vi "Post_Process_Raw_data.vi"(0 "Select Plug Ins":bool, 2 "Post processed Results folder":path, 3 "No dialogs":bool, 5 "Save results to":T1(ring)=enum."Original Results Filenames with _PP", 11 "Selected files":path[](array[path]), 12 "Current Results filenames":path[](array[path]), 13 "Results Plotter Rows":string[][](array[string])) -> (15 "Post processed Results folder Out":path)   [LabVIEW 2013]
uses:
  Anemometry Sub Vis/Controls/File_Selector_Type.ctl
  Anemometry Sub Vis/Controls/Setup.ctl
  Anemometry Sub Vis/Controls/Post_Process.ctl
  Anemometry Sub Vis/Controls/Save_Data.ctl
  Anemometry Sub Vis/Globals/Meas_global.vi
  Anemometry Sub Vis/Globals/Plug_in_data_global.vi
panel:
  out "Single Filename":string
  out "Files not found":i32
  out "Files not Found":path[](array[path])
  out "Checking":i32
  in  "Previous Choice":path
  in  "Search String":string
  in  "Boolean":bool
  in  "Pause Mode":enum16{"Continuous Running", "After Each File"}(ring)
  in  "At Dialog Prompt Post Process":T2=enum."All files listed in selected file"
  out "Files Processed":i32(slide) scale=0.0..253.0
  in  "stop":bool
  out "Files To Process":path[](array[path])
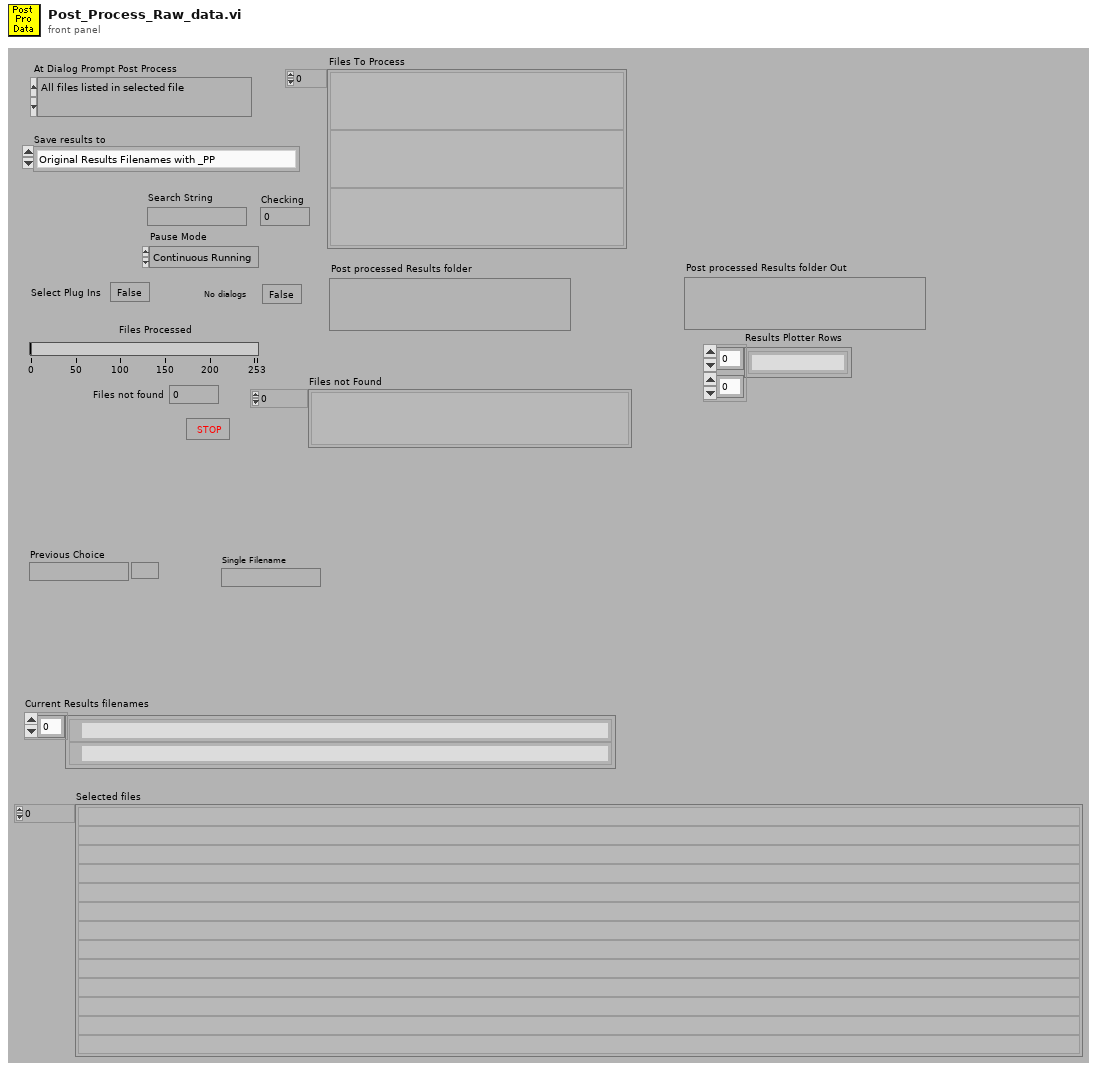
[diagram p1: front panel]
types:
  T1 = enum16{"A single file", "Original Results Filenames with _PP", "Current Results Filenames"}
  T2 = typedef "File_Selector_Type.ctl" = enum16{"The Selected File", "The Selected Folder", "Files containing the search string in the selected folder", "All files listed in selected file"}
  T3 = typedef "Setup.ctl" = enum16{"Run Program", "Show Setup", "Save Current Setup", "Setup Front Panel"}
  T4 = typedef "Save_Data.ctl" = enum16{"Save No Data", "Save Data"}
  T5 = typedef "Post_Process.ctl" = enum16{"Take New Data", "Post Process Raw Data File"}
  T6 = enum16{"Left Button", "Center Button", "Right Button", "Window Close"}
  T7 = typedef "Multi_Run_Status.ctl" = enum16{"Continue", "Jump to Next Point", "Jump to Next Row", "Jump To Fall Back", "Terminate Run"}
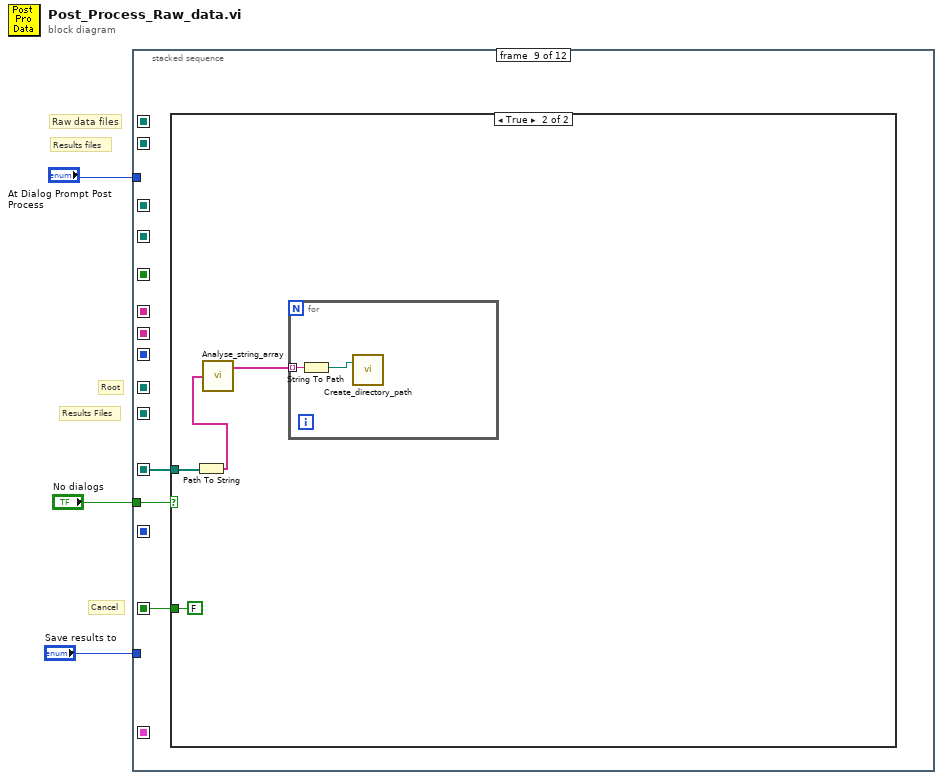
[diagram p0: block diagram]
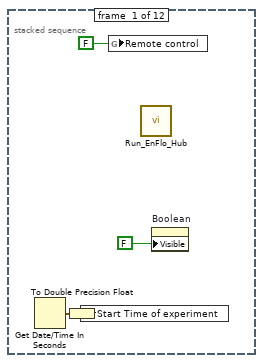
[diagram p2: hidden frame]
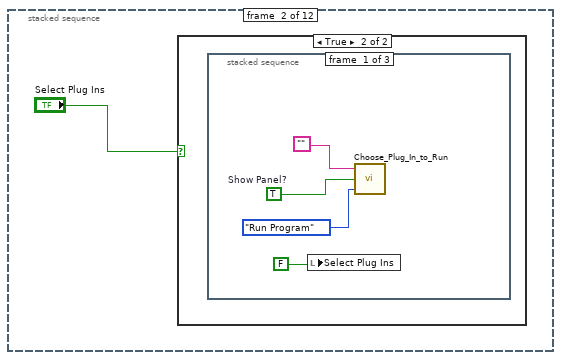
[diagram p3: hidden frame]
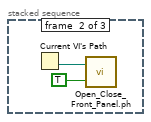
[diagram p5: hidden frame]
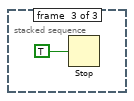
[diagram p6: hidden frame]
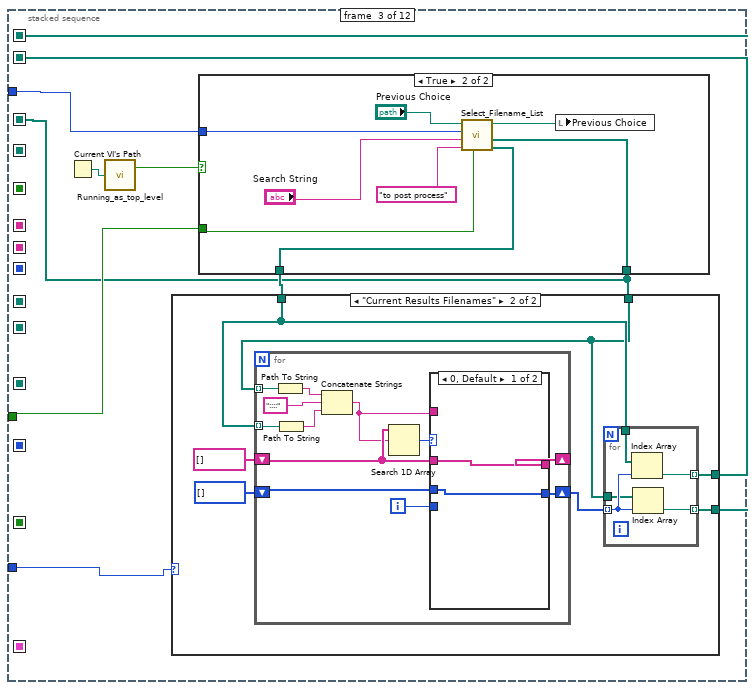
[diagram p7: hidden frame]
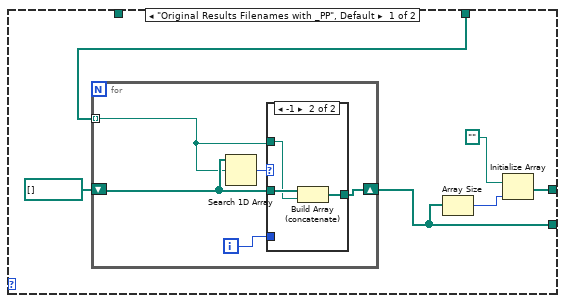
[diagram p8: hidden frame]
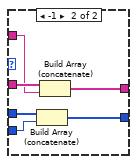
[diagram p10: hidden frame]
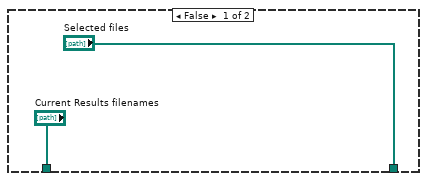
[diagram p11: hidden frame]
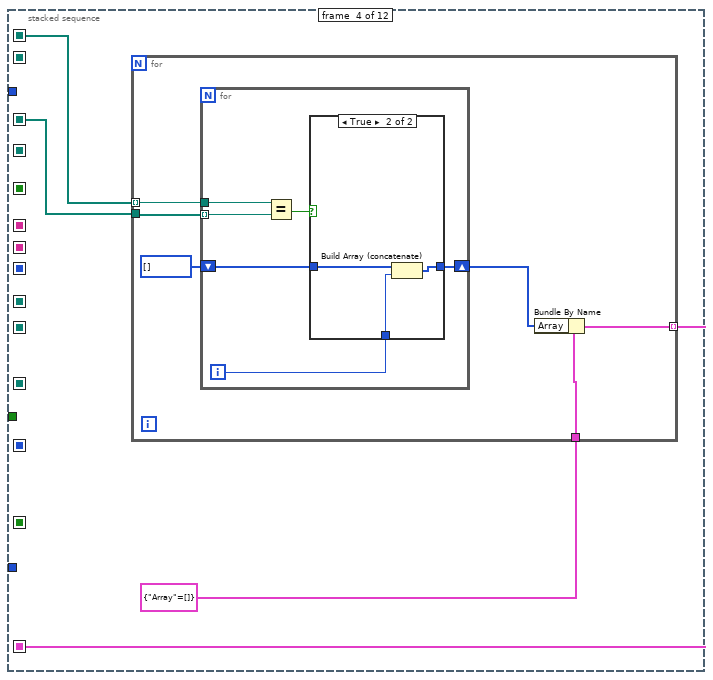
[diagram p12: hidden frame]
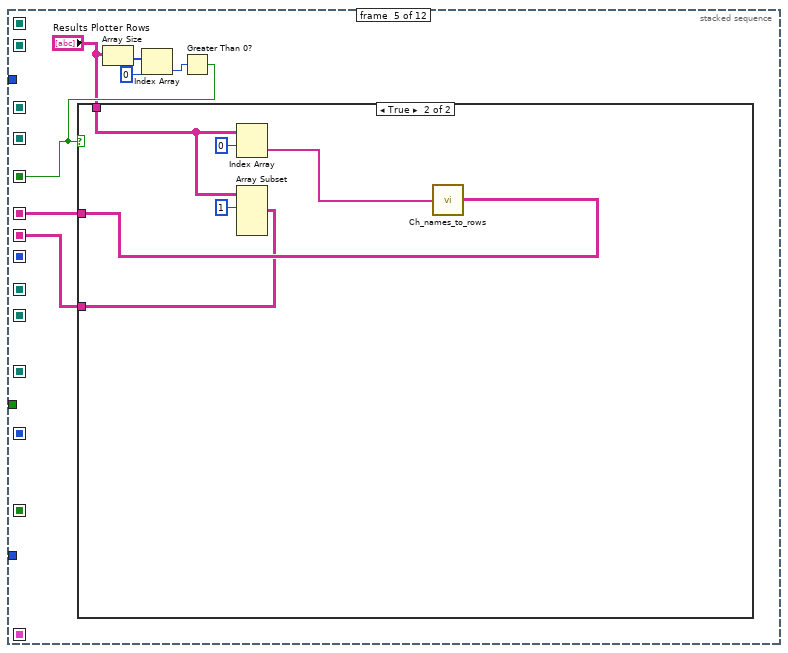
[diagram p14: hidden frame]
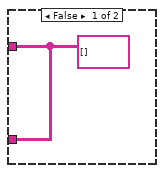
[diagram p15: hidden frame]
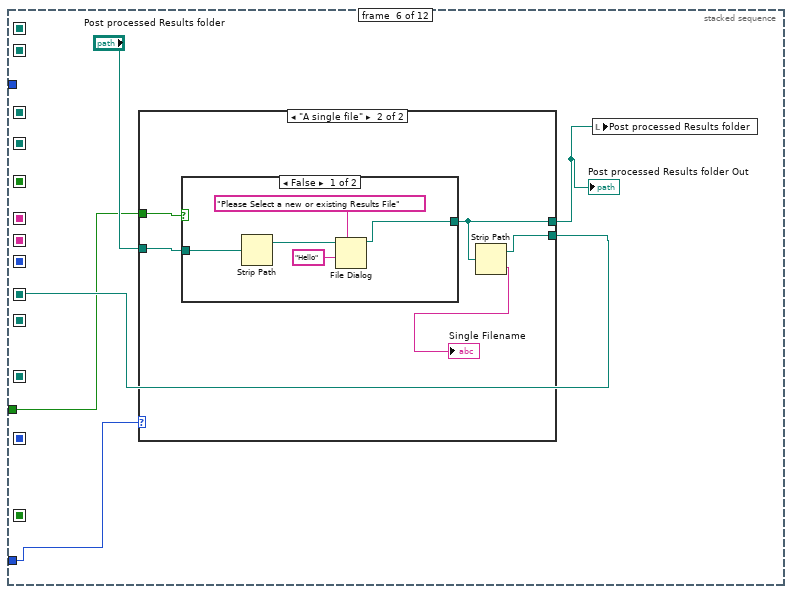
[diagram p16: hidden frame]
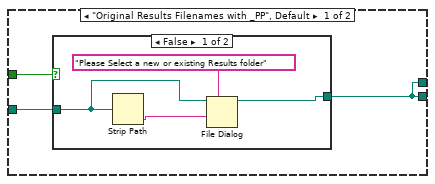
[diagram p17: hidden frame]
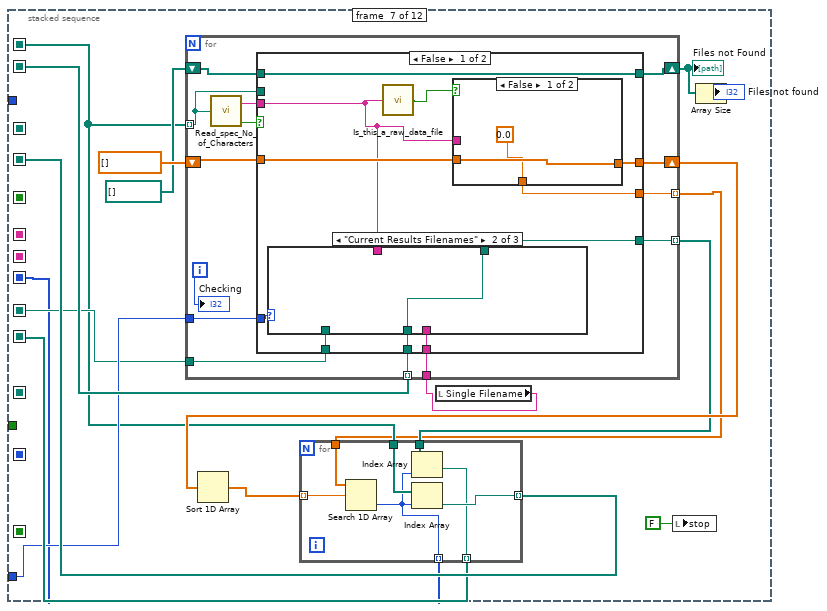
[diagram p20: hidden frame]
diagram:
  # "Cancel"
  # "Results files"
  # "Raw data files"
  # "Root"
  # "Results Files"
  n1 = stacked-sequence {
    seq-local: [_ _ _ _ _ _ w153 _ _ _ _ _] -> [_ _ _ _ _ _ _ _ _ w283 w297 _]
    seq-local: [_ _ _ _ _ _ _ _ _ w288 _ _] -> [_ _ _ _ _ _ _ _ _ _ w296 _]
    seq-local: [_ _ w18 _ _ _ _ _ _ _ _ _] -> [_ _ _ w84 _ _ w142 _ _ _ _ _]
    seq-local: [_ _ _ _ _ w120 _ _ _ _ _ _] -> [_ _ _ _ _ _ w145 w212 _ _ _ _]
    seq-local: [_ _ _ _ _ _ w151 _ _ _ _ _] -> [_ _ _ _ _ _ _ w215 _ _ _ _]
    seq-local: [_ _ _ _ _ _ _ w211 _ _ _ _] -> [_ _ _ _ _ _ _ _ w255 _ w295 w368]
    seq-local: [_ _ w19 _ _ _ _ _ _ _ _ _] -> [_ _ _ _ _ _ w147 _ _ _ _ _]
    seq-local: [_ _ _ _ w108 _ _ _ _ _ _ _] -> [_ _ _ _ _ _ _ _ _ _ w294 _]
    seq-local: [_ _ _ _ w107 _ _ _ _ _ _ _] -> [_ _ _ _ _ _ _ _ _ _ w291 _]
    seq-local: [_ _ _ _ w103 _ _ _ _ _ _ _] -> [_ _ _ _ _ _ _ _ _ _ w293 _]
    seq-local: [_ _ _ _ _ _ w143 _ _ _ _ _] -> [_ _ _ _ _ _ _ _ _ _ w292 _]
    seq-local: [_ _ _ w82 _ _ _ _ _ _ _ _] -> [_ _ _ _ _ _ _ _ _ _ w290 _]
    seq-local: [_ _ w16 _ _ _ _ _ _ _ _ _] -> [_ _ _ w85 _ _ _ _ _ _ _ _]
    seq-local: [_ _ _ _ _ _ _ _ w254 _ _ _] -> [_ _ _ _ _ _ _ _ _ _ w289 _]
    tunnel: "At Dialog Prompt Post Process" -> [_ _ w24 _ _ _ _ _ _ _ _ _]
    tunnel: "No dialogs" -> [_ _ w23 _ _ w118 _ _ w256 _ _ _]
    tunnel: "Save results to" -> [_ _ w17 _ _ w117 w146 w214 _ _ _ _]
    frame #0 {
      n2 = Get Date/Time In Seconds() -> (seconds since 1Jan1904=w4:timestamp)
      n3 = To Double Precision Float(number=w4) -> (double precision float=w5:dbl)
      n4 = global write "Meas_global.vi" "Start Time of experiment"(w5) -> ()
      n5 = global write "Meas_global.vi" "Remote control"(FALSE ("Remote control")) -> ()
      n6 = call "Run_EnFlo_Hub.vi"() -> ()  [unwired: 8 out]
      n7 = property on="Boolean" class="Bool"("Visible"=FALSE ("Write Attribute")) -> ()  [unwired: 2 in, 2 out]
    }
    frame #1 {
      n8 = case shown="True" "Select Plug Ins" {
        frame False {
        }
        frame True {
          n9 = stacked-sequence {
            frame #0 {
              w12 = TRUE  # Show Panel?
              n10 = local write "Select Plug Ins"(FALSE ("Select Local ADAM Channels")) -> ()
              n11 = call "Choose_Plug_In_to_Run.vi"("setup"=Setup."Run Program", "Show Panel?"=w12, "Setup String In"="") -> ()  [unwired: 2 out]
            }
            frame #1 {
              n12 = Current VI's Path() -> (path=w14:path)
              n13 = call "Open_Close_Front_Panel.ph.vi"("Front Panel Window:Open"=TRUE, "VI path"=w14) -> ()  [unwired: 2 out]
            }
            frame #2 {
              n14 = Stop(stop? (T)=TRUE) -> ()
            }
          }
        }
      }
    }
    frame #2 {
      n15 = Current VI's Path() -> (path=w22:path)
      n16 = call "Running_as_top_level.vi"("Vi path name"=w22) -> ("Top Level"=w21:bool)  [unwired: 1 out]
      n17 = case shown="True" w21 {
        tunnel: w24 -> [_ w81]
        tunnel: w23 -> [_ w76]
        tunnel: ["Selected files" w75] -> w16
        tunnel: ["Current Results filenames" w74] -> w20
        frame False {
        }
        frame True {
          n18 = call "Select_Filename_List.vi"("No dialogs"=w76, "File Type"="to post process", "Search String"="Search String", "At Dialog Prompt Post Process"=w81, "Previous Choice"="Previous Choice") -> ("Current Results filenames"=w74:path[], "Selected files"=w75:path[], "Choosen path"=w77:path)  [unwired: 1 out]
          n19 = local write "Previous Choice"(w77) -> ()
        }
      }
      n20 = case shown="\"Current Results Filenames\"" w17 {
        tunnel: w16 -> [w30 w43]
        tunnel: w20 -> [_ w44]
        tunnel: [w26 w42] -> w19
        tunnel: [w28 w41] -> w18
        frame "Original Results Filenames with _PP", Default {
          n21 = for {
            shift-right: [w34] -> w28
            shift-left: path[] [] -> [w35]
            tunnel: w30 -> [w31] mode=indexing
            i -> [w32]
            n22 = Search 1D Array(1D array=w35, element=w31) -> (index of element=w33:i32)  [unwired: 1 out]
            n23 = case shown="-1" w33 {
              tunnel: w35 -> [w36 w39]
              tunnel: [w36 w38] -> w34
              tunnel: w31 -> [_ w37]
              tunnel: w32 -> [_ _]
              frame 0, Default {
              }
              frame -1 {
                n24 = Build Array (concatenate)(w39, w37) -> (w38:path[])
              }
            }
          }
          n25 = Array Size(array=w28) -> (size(s)=w27:i32)
          n26 = Initialize Array(path "", w27) -> (w26:path[])
        }
        frame "Current Results Filenames" {
          n27 = for {
            shift-right: [w62] -> _
            shift-left: string[] [] -> [w63]
            tunnel: w43 -> [w61] mode=indexing
            tunnel: w44 -> [w55] mode=indexing
            shift-right: [w57] -> w40
            shift-left: i32[] [] -> [w56]
            i -> [w58]
            n28 = Path To String(path=w61) -> (string=w60:string)
            n29 = Path To String(path=w55) -> (string=w54:string)
            n30 = Concatenate Strings(w60, "::::" ("string"), w54) -> (w53:string)
            n31 = Search 1D Array(1D array=w63, element=w53) -> (index of element=w52:i32)  [unwired: 1 out]
            n32 = case shown="0, Default" w52 {
              tunnel: w63 -> [w65 w71]
              tunnel: [w65 w70] -> w62
              tunnel: w53 -> [_ w67]
              tunnel: w58 -> [_ w66]
              tunnel: [w64 w69] -> w57
              tunnel: w56 -> [w64 w68]
              frame 0, Default {
              }
              frame -1 {
                n33 = Build Array (concatenate)(w68, w66) -> (w69:i32[])
                n34 = Build Array (concatenate)(w71, w67) -> (w70:string[])
              }
            }
          }
          n35 = for {
            tunnel: w40 -> [w51] mode=indexing
            tunnel: w44 -> [w50]
            tunnel: w43 -> [w49]
            tunnel: [w48] -> w42 mode=indexing
            tunnel: [w47] -> w41 mode=indexing
            n36 = Index Array(array=w50, index=w51) -> (element=w48:path)
            n37 = Index Array(array=w49, index=w51) -> (element=w47:path)
          }
        }
      }
    }
    frame #3 {
      n38 = for {
        tunnel: w85 -> [w90]
        tunnel: w84 -> [w91] mode=indexing
        tunnel: cluster{"Array":i64[]} {"Array"=[]} ("Cluster") -> [w88]
        tunnel: [w86] -> w82 mode=indexing
        n39 = for {
          tunnel: w91 -> [w97]
          tunnel: w90 -> [w96] mode=indexing
          shift-right: [w93] -> w87
          shift-left: i32[] [] -> [w94]
          i -> [w92]
          n40 = Equal?(x=w97, y=w96) -> (x = y?=w95:bool)
          n41 = case shown="True" w95 {
            tunnel: w94 -> [w98 w101]
            tunnel: [w98 w100] -> w93
            tunnel: w92 -> [_ w99]
            frame False {
            }
            frame True {
              n42 = Build Array (concatenate)(w101, w99) -> (w100:i32[])
            }
          }
        }
        n43 = Bundle By Name(cluster=w88, "Array"=w87) -> (w86:cluster{"Array":i64[]})
      }
    }
    frame #4 {
      n44 = Array Size(array="Results Plotter Rows") -> (size(s)=w106:i32[])
      n45 = Index Array(array=w106, index=0) -> (element=w104:i32)
      n46 = Greater Than 0?(x=w104) -> (x > 0?=w103:bool)
      n47 = case shown="True" w103 {
        tunnel: [w109 w115] -> w108
        tunnel: [w109 w110] -> w107
        tunnel: "Results Plotter Rows" -> [_ w113]
        frame False {
          w109 = string[][] [] ("3 Row names")
        }
        frame True {
          n48 = Index Array(array=w113, index (row)=0 ("index")) -> (element=w111:string[])  [unwired: 1 in]
          n49 = Array Subset(array=w113, index (row)=1 ("index")) -> (w110:string[][])  [unwired: 3 in]
          n50 = call "Ch_names_to_rows.vi"("Channel Names"=w111) -> ("3 Row names"=w115:string[][])
        }
      }
    }
    frame #5 {
      n51 = case shown="\"A single file\"" w117 {
        tunnel: [w121 w130] -> w120
        tunnel: "Post processed Results folder" -> [w123 w133]
        tunnel: w118 -> [w122 w132]
        tunnel: [w121 w131] -> w116
        frame "Original Results Filenames with _PP", Default {
          n52 = case shown="False" w122 {
            tunnel: [w127 w128] -> w121
            tunnel: w123 -> [w124 w128]
            frame False {
              n53 = Strip Path(path=w124) -> (name=w125:string)  [unwired: 1 out]
              n54 = File Dialog(7:"Please Select a new or existing Results folder" ("prompt"), 9:w125, 11:w124) -> (3:w127:path)  [unwired: 1 in, 6 out]
            }
            frame True {
            }
          }
        }
        frame "A single file" {
          n55 = case shown="False" w132 {
            tunnel: w133 -> [w137 w139]
            tunnel: [w136 w139] -> w131
            frame False {
              n56 = Strip Path(path=w137) -> (stripped path=w135:path)  [unwired: 1 out]
              n57 = File Dialog(7:"Please Select a new or existing Results File" ("prompt"), 9:"Hello" ("default name"), 11:w135) -> (3:w136:path)  [unwired: 1 in, 6 out]
            }
            frame True {
            }
          }
          n58 = Strip Path(path=w131) -> (stripped path=w130:path, name=→"Single Filename":string)
        }
      }
      "Post processed Results folder Out" <- w116
      n59 = local write "Post processed Results folder"(w116) -> ()
    }
    frame #6 {
      n60 = local read "Single Filename"() -> (w144:string)
      n61 = for {
        tunnel: w142 -> [w172] mode=indexing
        shift-right: [w176] -> w156
        shift-left: dbl[] [] -> [w177]
        shift-right: [w173] -> w149
        shift-left: path[] [] -> [w174]
        tunnel: w147 -> [w169] mode=indexing
        tunnel: w146 -> [w168]
        tunnel: w145 -> [w167]
        tunnel: w144 -> [w166]
        tunnel: [w165] -> w141 mode=indexing
        tunnel: [w164] -> w140 mode=indexing
        i -> [w175]
        n62 = call "Read_spec_No_of_Characters.vi"("Filename"=w172) -> ("character string"=w171:string, "Error?"=w170:bool)
        n63 = case shown="False" w170 {
          tunnel: w177 -> [w188 w210]
          tunnel: [w187 w210] -> w176
          tunnel: w172 -> [_ w208]
          tunnel: w174 -> [w185 w209]
          tunnel: [w185 w207] -> w173
          tunnel: w171 -> [w184 _]
          tunnel: w169 -> [w182 w206]
          tunnel: w168 -> [w183 _]
          tunnel: w167 -> [w181 _]
          tunnel: w166 -> [w180 _]
          tunnel: [w179 w206] -> w165
          tunnel: [w178 0.0 ("Value")] -> w164
          frame False {
            n64 = case shown="\"Current Results Filenames\"" w183 {
              tunnel: [w191 w192 w195] -> w179
              tunnel: w184 -> [_ _ w193]
              tunnel: w182 -> [_ w192 _]
              tunnel: w181 -> [w190 _ _]
              tunnel: w180 -> [w189 _ _]
              frame "A single file" {
                n65 = Build Path(base path=w190, name or relative path=w189) -> (appended path=w191:path)
              }
              frame "Current Results Filenames" {
              }
              frame "Original Results Filenames with _PP" {
                w196 = FALSE  # Show Dialog?
                n66 = call "Get_Characters_from_string.vi"("Show Dialog?"=w196, "Input string"=w193, "Variable name"="Results filename") -> ("Value"=w194:string)  [unwired: 1 out]
                n67 = call "String_to_Pathname.vi"("Input String"=w194) -> ("path"=w195:path)
              }
            }
            n68 = call "Is_this_a_raw_data_file.vi"("character string"=w184) -> ("Raw Dat File?"=w186:bool)  [unwired: 2 out]
            n69 = case shown="False" w186 {
              tunnel: w188 -> [w199 w201]
              tunnel: [w199 w204] -> w187
              tunnel: w184 -> [_ w202]
              tunnel: [0.0 ("Value") w200] -> w178
              frame False {
              }
              frame True {
                n70 = call "Get_value_from_string.vi"("Input string"=w202, "Variable name"="Seconds since 1/1/04") -> ("Value"=w200:dbl)  [unwired: 1 in, 1 out]
                n71 = Build Array (concatenate)(w201, w200) -> (w204:dbl[])
              }
            }
          }
          frame True {
            n72 = Build Array (concatenate)(w209, w208) -> (w207:path[])
          }
        }
        "Checking" <- w175
      }
      "Files not Found" <- w149
      n73 = Sort 1D Array(array=w156) -> (sorted array=w155:dbl[])
      n74 = for {
        tunnel: w140 -> [w163]
        tunnel: w155 -> [w162] mode=indexing
        tunnel: w142 -> [w161]
        tunnel: [w160] -> w153 mode=indexing
        tunnel: w141 -> [w159]
        tunnel: [w158] -> w151 mode=indexing
        tunnel: [w157] -> w143 mode=indexing
        n75 = Search 1D Array(1D array=w163, element=w162) -> (index of element=w157:i32)  [unwired: 1 out]
        n76 = Index Array(array=w159, index=w157) -> (element=w158:path)
        n77 = Index Array(array=w161, index=w157) -> (element=w160:path)
      }
      n78 = local write "stop"(FALSE ("stop")) -> ()
      n79 = Array Size(array=w149) -> (size(s)=→"Files not found":i32)
    }
    frame #7 {
      n80 = case shown="\"Original Results Filenames with _PP\"" w214 {
        tunnel: [FALSE TRUE] -> w213
        tunnel: w214 -> [_ _]
        frame "A single file", Default {
        }
        frame "Original Results Filenames with _PP" {
        }
      }
      n81 = for {
        tunnel: w215 -> [w249] mode=indexing
        tunnel: w213 -> [w221]
        tunnel: w212 -> [w220]
        tunnel: [w218] -> w211 mode=indexing
        w234 = "_" ("Replace with")
        n82 = Strip Path(path=w249) -> (name=w222:string)  [unwired: 1 out]
        n83 = Concatenate Strings("[" ("Substring"), ":", "/", "\\\\", "|", "?", ">", "<", "*", "\"", "]" ("Substring")) -> (w237:string)
        n84 = call <vilib>:"Trim Whitespace.vi"("string"=w222) -> ("trimmed string"=w236:string)  [unwired: 1 in]
        n85 = call "Add_filename_suffix.vi"("Filename"=w236) -> ("Original Suffix"=w226:string, "Base name"=w235:string)  [unwired: 1 in, 2 out]
        n86 = call "Replace_Character.vi"("Replace with"=w234, "Input String"=w235, "Search For"=w237) -> ("Output string"=w230:string)  [unwired: 1 out]
        n87 = call "Replace_Character.vi"("Replace with"="_", "Input String"=w230, "Search For"=" ") -> ("Output string"=w231:string)  [unwired: 1 out]
        n88 = case shown="False" w221 {
          tunnel: [w250 w252] -> w233
          tunnel: w231 -> [w250 w251]
          frame False {
          }
          frame True {
            n89 = Concatenate Strings(w251, "_pp" ("Substring")) -> (w252:string)
          }
        }
        n90 = Empty String/Path?(string/path=w226) -> (empty?=w227:bool)
        n91 = Select(t=".xls", s=w227, f=w226) -> (s? t:f=w225:string)
        n92 = call "Replace_Character.vi"("Replace with"=w234, "Input String"=w233, "Search For"="__") -> ("Output string"=w224:string)  [unwired: 1 out]
        n93 = Concatenate Strings(w224, w225) -> (w219:string)
        n94 = Build Path(base path=w220, name or relative path=w219) -> (appended path=w218:path)
      }
    }
    frame #8 {
      n95 = case shown="True" w256 {
        tunnel: w255 -> [w260 w278]
        tunnel: [w257 FALSE ("stop? (T)")] -> w254
        frame False {
          n96 = Path To String(path=w260) -> (string=w259:string[])
          n97 = call "Analyse_string_array.vi"("String array"=w259) -> ("Unique strings"=w258:string[])  [unwired: 2 out]
          n98 = for {
            tunnel: w258 -> [w263] mode=indexing
            tunnel: [w262] -> w257
            stop <- w262 stop-if-true
            n99 = String To Path(string=w263) -> (path=w261:path)
            n100 = call "Does_file_exist_(simple).vi"("Pathname"=w261) -> ("exists?"=w264:bool)
            n101 = call "Create_directory_path.vi"("Path name"=w261) -> ()  [unwired: 1 in, 2 out]
            n102 = case shown="True" w264 {
              tunnel: w261 -> [_ w267]
              tunnel: [FALSE ("stop? (T)") w266] -> w262
              frame False {
              }
              frame True {
                n103 = Format Into String(format string="%s\nAlready exists. Do you want to overwrite?", w267) -> (resulting string=w270:string)  [unwired: 2 in, 1 out]
                n104 = call <vilib>:"Three Button Dialog.vi"("Allow user to close window? (TRUE)"=FALSE, "message"=w270) -> ("Which Button?"=w268:T6)  [unwired: 9 in]
                n105 = case shown="\"Center Button\"" w268 {
                  tunnel: w267 -> [w273 _ _ _]
                  tunnel: [FALSE ("stop? (T)") FALSE ("stop? (T)") TRUE ("stop? (T)") FALSE ("stop? (T)")] -> w266
                  frame "Left Button" {
                    n106 = Delete(path (use dialog)=w273) -> ()  [unwired: 4 in, 3 out]
                  }
                  frame "Center Button" {
                  }
                  frame "Right Button" {
                  }
                  frame "Window Close" {
                  }
                }
              }
            }
          }
        }
        frame True {
          n107 = Path To String(path=w278) -> (string=w279:string[])
          n108 = call "Analyse_string_array.vi"("String array"=w279) -> ("Unique strings"=w277:string[])  [unwired: 2 out]
          n109 = for {
            tunnel: w277 -> [w282] mode=indexing
            n110 = String To Path(string=w282) -> (path=w281:path)
            n111 = call "Create_directory_path.vi"("Path name"=w281) -> ()  [unwired: 1 in, 2 out]
          }
        }
      }
    }
    frame #9 {
      w284 = 0 ("Files Processed")
      n112 = Array Size(array=w283) -> (size(s)=w288:i32)
      n113 = Array Size(array=w283) -> (size(s)=w286:i32)
      n114 = property on="Files Processed" class="Slide (strict)"("Scale.Range:Minimum"=0.0 ("Write Attribute"), "Scale.Range:Maximum"=w286) -> ()  [unwired: 2 in, 2 out]
      n115 = local write "Files Processed"(w284) -> ()
      n116 = Build Array(w284) -> (w285:i32[])
      n117 = property on="Attribute Node" class="Arr (strict)"("Index Values"=w285) -> ()  [unwired: 2 in, 2 out]
      "Files To Process" <- w283
    }
    frame #10 {
      n118 = case shown="False" w289 {
        tunnel: w297 -> [w305 _]
        tunnel: w296 -> [w304 _]
        tunnel: w295 -> [w303 _]
        tunnel: w294 -> [w302 _]
        tunnel: w293 -> [w301 _]
        tunnel: w292 -> [w300 _]
        tunnel: w291 -> [w299 _]
        tunnel: w290 -> [w298 _]
        frame False {
          n119 = while {
            tunnel: w303 -> [w311] mode=indexing
            tunnel: w304 -> [w314]
            tunnel: w305 -> [w315] mode=indexing
            tunnel: w302 -> [w310]
            tunnel: w300 -> [w307] mode=indexing
            tunnel: w301 -> [w309]
            tunnel: w299 -> [w308]
            tunnel: w298 -> [w306]
            i -> [w313]
            stop <- w312 continue-if-true
            n120 = stacked-sequence {
              seq-local: [_ w337 _ _] -> [_ _ w341 _]
              tunnel: w311 -> [_ w339 _ _]
              tunnel: w315 -> [_ w338 _ _]
              tunnel: w314 -> [_ _ w343 _]
              tunnel: w313 -> [_ _ w342 w365]
              tunnel: [_ _ w340 _] -> w312
              tunnel: w310 -> [w324 _ _ _]
              tunnel: w309 -> [w323 _ _ _]
              tunnel: w308 -> [w319 _ _ _]
              tunnel: w307 -> [w320 _ _ _]
              tunnel: w306 -> [w321 _ _ _]
              frame #0 {
                n121 = Index Array(array=w321, index=w320) -> (element=w318:cluster{"Array":i64[]})
                n122 = Unbundle By Name(w318) -> ("Array"=w317:i64[])
                n123 = for {
                  tunnel: w319 -> [w327]
                  tunnel: w317 -> [w326] mode=indexing
                  tunnel: [w325] -> w316 mode=indexing
                  n124 = Index Array(array=w327, index (row)=w326) -> (element=w325:string[])  [unwired: 1 in]
                }
                n125 = case shown="True" w323 {
                  tunnel: w324 -> [_ w331]
                  tunnel: w316 -> [_ w330]
                  tunnel: ["" w329] -> w322
                  frame False {
                  }
                  frame True {
                    n126 = Build Array (concatenate)(w331, w330) -> (w333:string[][])
                    n127 = Array To Spreadsheet String(array=w333, 3:"%s" ("format string")) -> (spreadsheet string=w329:string)  [unwired: 1 out]
                  }
                }
                n128 = global write "Plug_in_data_global.vi" "Templated Results header"(w322) -> ()
              }
              frame #1 {
                n129 = call "Measurement.vi"("setup"=Setup."Run Program", "Post Process"=Post_Process."Post Process Raw Data File", "File"=Save_Data."Save Data", "Results file"=w339, "Raw data file"=w338) -> ("Status Out"=w337:T7)  [unwired: 2 in, 12 out]
              }
              frame #2 {
                n130 = Increment(x=w342) -> (x+1=w345:i32)
                n131 = Less?(x=w345, y=w343) -> (x < y?=w344:bool)
                n132 = while {
                  shift-left: _ -> [w351]
                  shift-right: [w352] -> _
                  tunnel: [w354] -> w340
                  tunnel: w341 -> [w355]
                  tunnel: w344 -> [w347]
                  stop <- w350 continue-if-true
                  n133 = case shown="\"After Each File\"" "Pause Mode" {
                    tunnel: [TRUE "Boolean"] -> w349
                    tunnel: w351 -> [_ w360]
                    frame "Continuous Running" {
                    }
                    frame "After Each File" {
                      n134 = Select(t=u32 500 ("milliseconds to wait"), s=w360, f=u32 100) -> (s? t:f=w357:u32)
                      n135 = property on="Boolean" class="Bool"("Visible"=w360, "Key Focus"=w360) -> ()  [unwired: 2 in, 2 out]
                      n136 = Wait (ms)(milliseconds to wait=w357) -> ()  [unwired: 1 out]
                    }
                  }
                  n137 = Compound Arithmetic op=AND(invert w349, invert "stop", w347) -> (w350:bool)
                  n138 = Compound Arithmetic op=AND(w349, invert "stop", w347) -> (w346:bool)
                  n139 = case shown="\"Continue\", Default" w355 {
                    tunnel: [w362 FALSE] -> w354
                    tunnel: w346 -> [w362 _]
                    frame "Continue", Default {
                    }
                    frame "Terminate Run" {
                    }
                  }
                  n140 = Not(x=w351) -> (.not. x?=w352:bool)
                }
              }
              frame #3 {
                n141 = Increment(x=w365) -> (x+1=w364:i32)
                "Files Processed" <- w364
                n142 = Build Array(w364) -> (w366:i32[])
                n143 = property on="Attribute Node" class="Arr (strict)"("Index Values"=w366) -> ()  [unwired: 2 in, 2 out]
              }
            }
          }
        }
        frame True {
        }
      }
    }
    frame #11 {
      n144 = Path To String(path=w368) -> (string=w370:string[])
      n145 = call "Analyse_string_array.vi"("String array"=w370) -> ("Unique strings"=w369:string[])  [unwired: 2 out]
      n146 = String To Path(string=w369) -> (path=w367:path[])
      n147 = for {
        tunnel: w367 -> [w374] mode=indexing
        w375 = FALSE  # Lock File
        n148 = call "Lock_File.vi"("Lock File"=w375, "path"=w374) -> ()  [unwired: 1 in, 3 out]
      }
      n149 = Build Array(0) -> (w372:i32[])
      n150 = property on="Boolean" class="Bool"("Visible"=FALSE ("Write Attribute")) -> ()  [unwired: 2 in, 2 out]
      n151 = property on="Attribute Node" class="Arr (strict)"("Index Values"=w372) -> ()  [unwired: 2 in, 2 out]
    }
  }
